vi "Write Avg to File.vi"(8 "error in":errorcluster) -> (0 "error out":errorcluster)   [LabVIEW 2017, in "Akwizycja.lvlib"]
uses:
  Akwizycja.lvlib
panel:
  in  "output cluster":T1
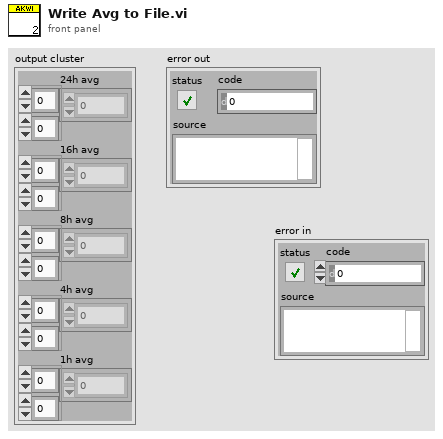
[diagram p1: front panel]
types:
  T1 = cluster{"24h avg":dbl[][], "16h avg":dbl[][], "8h avg":dbl[][], "4h avg":dbl[][], "1h avg":dbl[][]}
  T2 = enum16{"open", "replace", "create", "open or create", "replace or create", "replace or create with confirmation"}
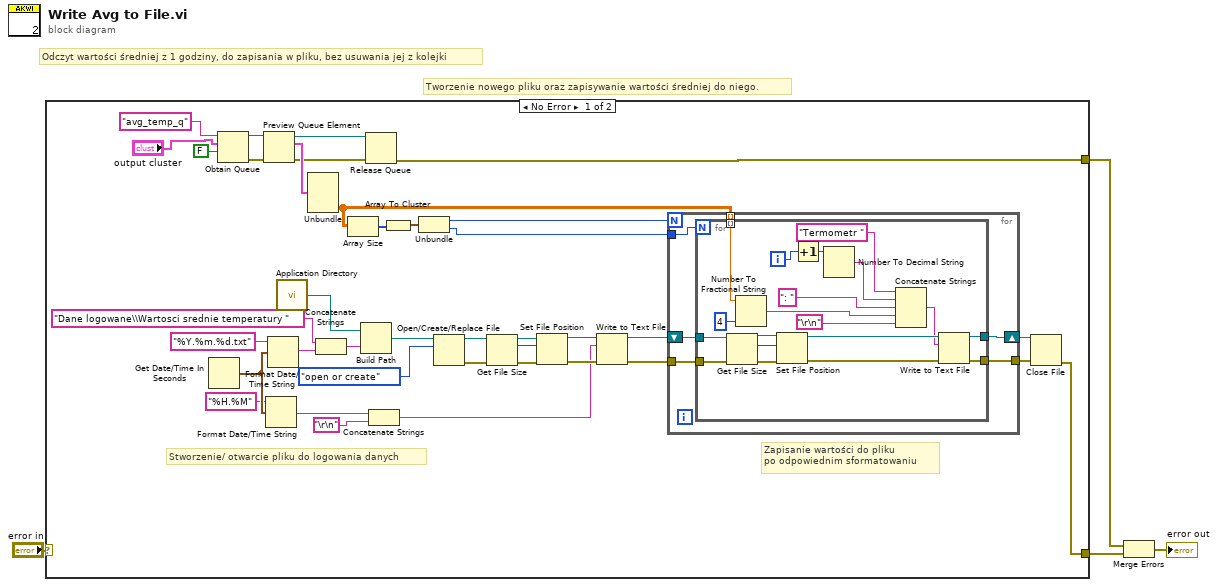
[diagram p0: block diagram]
diagram:
  # "Odczyt wartości średniej z 1 godziny, do zapisania w pliku, bez usuwania jej z kolejki"
  # "Tworzenie nowego pliku oraz zapisywanie wartości średniej do niego."
  n1 = case shown="No Error" "error in" {
    selector: "error in" -> [_ w68]
    tunnel: [w11 w68] -> w2
    tunnel: [w21 _] -> w1
    frame No Error {
      # "Zapisanie wartości do pliku\npo odpowiednim sformatowaniu"
      # "Stworzenie/ otwarcie pliku do logowania danych"
      n2 = Get Date/Time In Seconds() -> (seconds since 1Jan1904=w10:timestamp)
      n3 = Obtain Queue(name (unnamed)="avg_temp_q", element data type="output cluster", create if not found? (T)=FALSE) -> (queue out=w22:refnum<queue>, error out=w26:errorcluster)  [unwired: 2 in, 1 out]
      n4 = Preview Queue Element(queue=w22, error in (no error)=w26) -> (queue out=w25:refnum<queue>, element=w29:T1, error out=w27:errorcluster)  [unwired: 1 in, 1 out]
      n5 = Format Date/Time String(time format string (%c)="%H.%M", seconds (now)=w10) -> (date/time string=w7:string)  [unwired: 1 in]
      n6 = Format Date/Time String(time format string (%c)="%Y.%m.%d.txt", seconds (now)=w10) -> (date/time string=w32:string)  [unwired: 1 in]
      n7 = call <vilib>:"Application Directory.vi"() -> ("Application Directory"=w33:path)
      n8 = Unbundle(w29) -> ("1h avg"=w38:dbl[][])  [unwired: 4 out]
      n9 = Concatenate Strings("Dane logowane\\Wartosci srednie temperatury " ("name or relative path"), w32) -> (w34:string)
      n10 = Array Size(array=w38) -> (size(s)=w39:i32[])
      n11 = Build Path(base path=w33, name or relative path=w34) -> (appended path=w36:path)
      n12 = Release Queue(queue=w25, error in (no error)=w27) -> (error out=w21:errorcluster)  [unwired: 1 in, 2 out]
      n13 = Concatenate Strings(w7, "\r\n") -> (w5:string)
      n14 = Array To Cluster(array=w39) -> (cluster=w40:cluster{"[0]":i32, "[1]":i32})
      n15 = Unbundle(w40) -> ("[0]"=w41:i32, "[1]"=w42:i32)
      n16 = Open/Create/Replace File(file path (use dialog)=w36, operation (0:open)=T2."open or create") -> (refnum out=w20:refnum<file>, error out=w19:errorcluster)  [unwired: 4 in, 1 out]
      n17 = Get File Size(file=w20, error in=w19) -> (refnum out=w16:refnum<file>, size (in bytes)=w8:i64, 0:w18:errorcluster)
      n18 = Set File Position(offset (in bytes) (0)=w8, refnum=w16, error in=w18) -> (refnum out=w15:refnum<file>, error out=w17:errorcluster)  [unwired: 1 in]
      n19 = Write to Text File(file (use dialog)=w15, text=w5, error in=w17) -> (refnum out=w14:refnum<file>, error out=w13:errorcluster)  [unwired: 1 in, 1 out]
      n20 = for {
        N: w41 -> [_]
        shift-right: [w47] -> w37
        shift-left: w14 -> [w48]
        tunnel: w38 -> [w46] mode=indexing
        tunnel: w42 -> [w45]
        tunnel: w13 -> [w44]
        tunnel: [w43] -> w12
        n21 = for {
          N: w45 -> [_]
          tunnel: w48 -> [w65]
          tunnel: [w64] -> w47
          tunnel: w46 -> [w51] mode=indexing
          tunnel: w44 -> [w62]
          tunnel: [w59] -> w43
          i -> [w57]
          n22 = Get File Size(file=w65, error in=w62) -> (refnum out=w67:refnum<file>, size (in bytes)=w66:i64, 0:w61:errorcluster)
          n23 = Number To Fractional String(number=w51, precision (6)=i16 4) -> (F-format string=w50:string)  [unwired: 2 in]
          n24 = Set File Position(offset (in bytes) (0)=w66, refnum=w67, error in=w61) -> (refnum out=w63:refnum<file>, error out=w60:errorcluster)  [unwired: 1 in]
          n25 = Increment(x=w57) -> (x+1=w56:i32)
          n26 = Number To Decimal String(number=w56) -> (decimal integer string=w54:string)  [unwired: 1 in]
          n27 = Concatenate Strings("Termometr ", w54, ": ", w50, "\r\n") -> (w58:string)
          n28 = Write to Text File(file (use dialog)=w63, text=w58, error in=w60) -> (refnum out=w64:refnum<file>, error out=w59:errorcluster)  [unwired: 1 in, 1 out]
        }
      }
      n29 = Close File(refnum=w37, error in=w12) -> (error out=w11:errorcluster)  [unwired: 1 out]
    }
    frame Error {
    }
  }
  n30 = Merge Errors(w1, w2) -> (→"error out":errorcluster)
